vi "GetDllPath.vi"() -> (0 "DllPath":path)   [LabVIEW 2018, in "ControlCan.lvlib"]
uses:
  ControlCan.lvlib
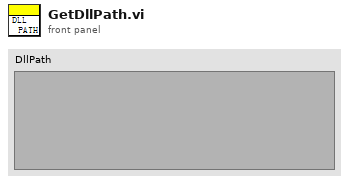
[diagram p1: front panel]
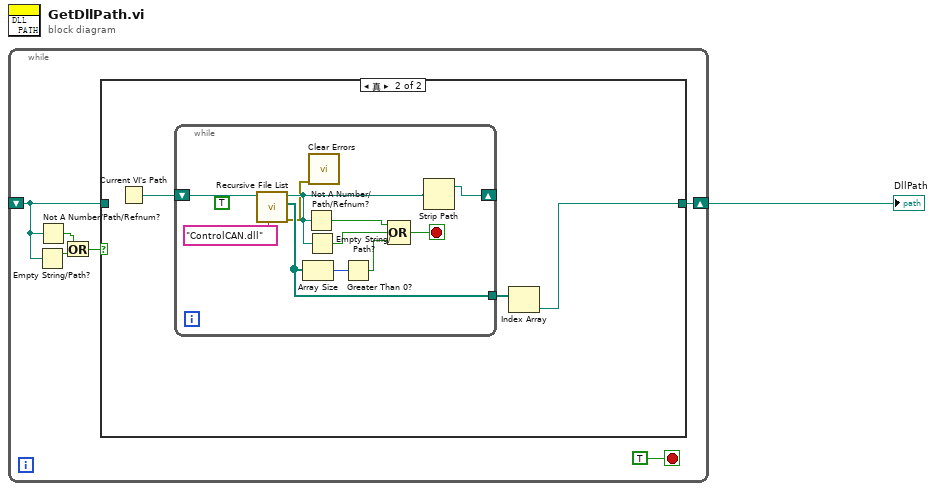
[diagram p0: block diagram]
diagram:
  n1 = while {
    shift-right: [w7] -> w1
    shift-left: _ -> [w2]
    stop <- TRUE stop-if-true
    n2 = Empty String/Path?(string/path=w2) -> (empty?=w4:bool)
    n3 = Not A Number/Path/Refnum?(number/path/refnum=w2) -> (NaN/Path/Refnum?=w5:bool)
    n4 = Or(x=w5, y=w4) -> (x .or. y?=w3:bool)
    n5 = case shown="真" w3 {
      tunnel: [w8 w10] -> w7
      tunnel: w2 -> [w8 _]
      frame False {
      }
      frame True {
        n6 = Current VI's Path() -> (path=w11:path)
        n7 = while {
          shift-right: [w14] -> _
          shift-left: w11 -> [w22]
          tunnel: [w13] -> w9
          stop <- w16 stop-if-true
          (unwired) TRUE ("Treat LLBs as Folders?")
          n8 = call <vilib>:"Recursive File List.vi"("pattern"="ControlCAN.dll", "Folder Path"=w22) -> ("error out"=w12:errorcluster, "All Files in Dir"=w13:path[], "dup Folder Path"=w15:path)  [unwired: 3 in, 4 out]
          n9 = Array Size(array=w13) -> (size(s)=w20:i32)
          n10 = Not A Number/Path/Refnum?(number/path/refnum=w15) -> (NaN/Path/Refnum?=w19:bool)
          n11 = Empty String/Path?(string/path=w15) -> (empty?=w18:bool)
          n12 = call <vilib>:"Clear Errors.vi"("error in (no error)"=w12) -> ()  [unwired: 1 in, 6 out]
          n13 = Greater Than 0?(x=w20) -> (x > 0?=w17:bool)
          n14 = Compound Arithmetic op=OR(w19, w18, w17) -> (w16:bool)
          n15 = Strip Path(path=w15) -> (stripped path=w14:path)  [unwired: 1 out]
        }
        n16 = Index Array(array=w9) -> (element=w10:path)  [unwired: 1 in]
      }
    }
  }
  "DllPath" <- w1
